vi "Generic Enum to String.vi"(8 "error in (no error)":errorcluster, 11 "Enum":variant) -> (0 "error out":errorcluster, 3 "EnumNames":string[](array[string]))   [LabVIEW 2011]
doc: "Converts a variant enum to a list if strings"
uses:
  <vilib>/Utility/VariantDataType/VariantType.lvlib
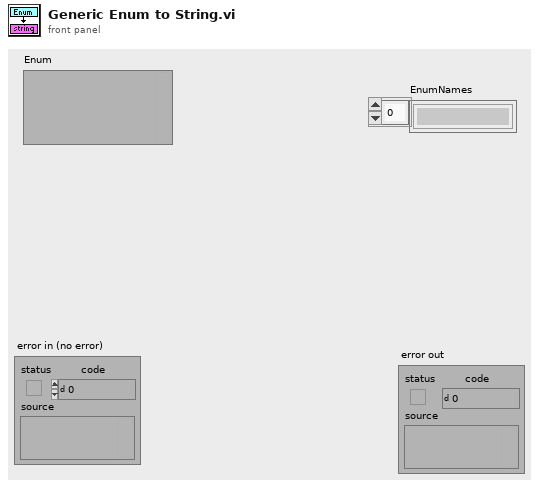
[diagram p1: front panel]
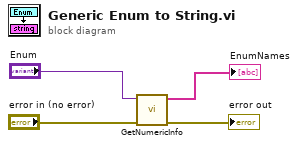
[diagram p0: block diagram]
diagram:
  n1 = call <vilib>:"GetNumericInfo.vi"("error in (no error)"="error in (no error)", "Variant"="Enum") -> ("error out"=→"error out":errorcluster, "EnumNames"=→"EnumNames":string[])  [unwired: 8 out]
